vi "GetBitfile.vi"(8 "error in (no error)":errorcluster, 11 "system info":T1) -> (0 "error out":errorcluster, 3 "Bitfile":path)   [LabVIEW 2017, in "McsaFpgaBitfileManager.lvlib"]
uses:
  <vilib>/addons/InsightCM/Devices/Shared/Mcsa/McsaFpgaBitfileManager/McsaFpgaBitfileManager.lvlib
  <vilib>/addons/cRIODetectHW/control/SystemHW.ctl
  <vilib>/addons/cRIODetectHW/control/cRIO Product Info.ctl
  <vilib>/addons/cRIODetectHW/cRIODetectHW.lvlib
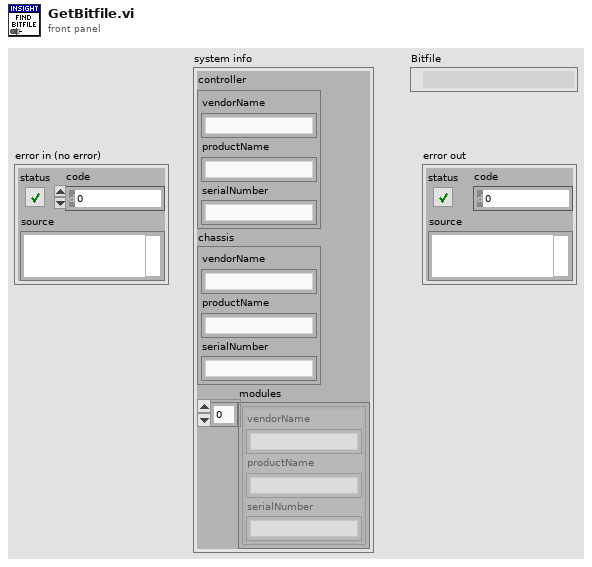
[diagram p1: front panel]
types:
  T1 = typedef "cRIODetectHW.lvlib/SystemHW.ctl" = cluster{"controller":T2, "chassis":T2, "modules":T2[]}
  T2 = typedef "cRIODetectHW.lvlib/cRIO Product Info.ctl" = cluster{"vendorName":string, "productName":string, "serialNumber":string}
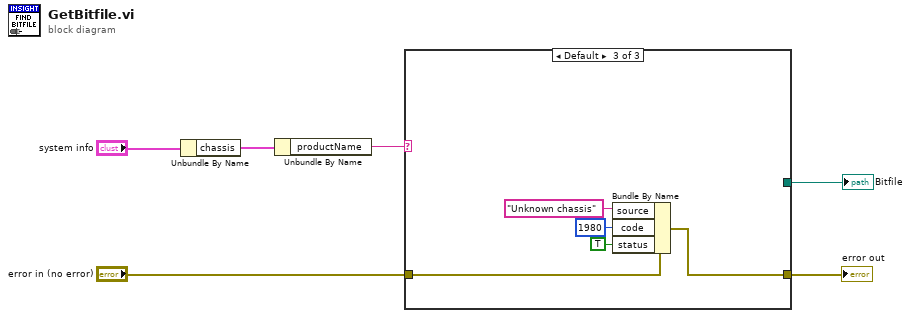
[diagram p0: block diagram]
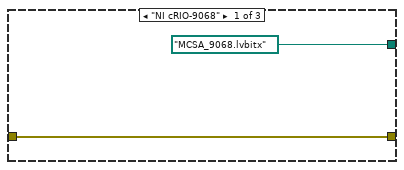
[diagram p2: hidden frame]
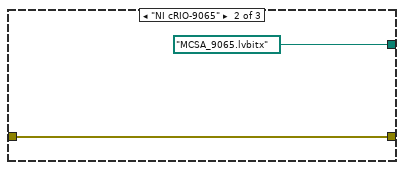
[diagram p3: hidden frame]
diagram:
  n1 = Unbundle By Name("system info") -> ("chassis"=w5:T2)
  n2 = Unbundle By Name(w5) -> ("productName"=w4:string)
  n3 = case shown="Default" w4 {
    tunnel: [path "MCSA_9068.lvbitx" path "MCSA_9065.lvbitx" _] -> w3
    tunnel: [w7 w9 w12] -> w2
    tunnel: "error in (no error)" -> [w7 w9 w13]
    frame "NI cRIO-9068" {
    }
    frame "NI cRIO-9065" {
    }
    frame Default {
      n4 = Bundle By Name(cluster=w13, "source"="Unknown chassis", "code"=1980, "status"=TRUE) -> (w12:errorcluster)
    }
  }
  "error out" <- w2
  "Bitfile" <- w3
